vi "Measure Lowlevel.vi"(0 "VISA resource name":refnum<visa-resource-name>, 1 "Buffer Elements":string="READ", 5 "Timeout (10000 ms)":i32=10000 format="%#.6g", 7 "Buffer Name (defbuffer1)":string="defbuffer1", 9 "Function (0: Volts)":u16(ring) items=["Volts", "Current", "Digitize Voltage", "Digitize Current"], 11 "error in (no error)":errorcluster) -> (4 "VISA resource name out":refnum<visa-resource-name>, 6 "Data out":string, 15 "error out":errorcluster)   [LabVIEW 2022 SP3, in "Keithley 2450.lvlib"]
doc: "Measures data for voltage, current and resistance. \n\nBuffer Element can be a single parameter or multiple parameters.Parameters have to be separated by comma followed by space.(eg - READ, SEC, DATE)"
uses:
  Keithley 2450.lvlib
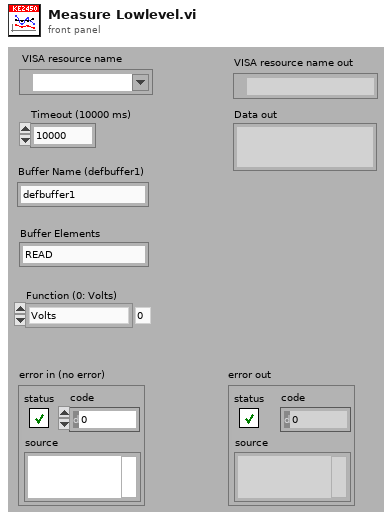
[diagram p1: front panel]
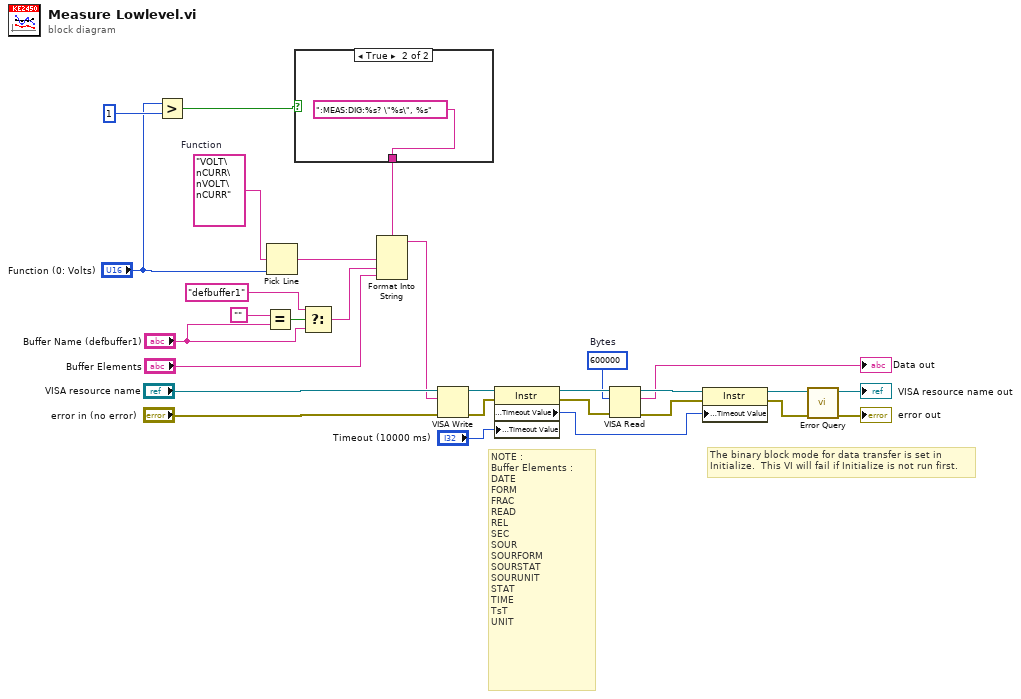
[diagram p0: block diagram]
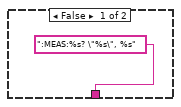
[diagram p2: hidden frame]
diagram:
  w9 = "VOLT\nCURR\nVOLT\nCURR"  # Function
  w20 = u32 600000  # Bytes
  # "NOTE :\nBuffer Elements :\nDATE\nFORM\nFRAC\nREAD\nREL\nSEC\nSOUR\nSOURFORM\nSOURSTAT\nSOURUNIT\nSTAT\nTIME\nTsT\nUNIT"
  # "The binary block mode for data transfer is set in Initialize.  This VI will fail if Initialize is not run first."
  n1 = Greater?(x="Function (0: Volts)", y=1) -> (0:w4:bool)
  n2 = Equal?(x="", y="Buffer Name (defbuffer1)") -> (x = y?=w16:bool)
  n3 = Pick Line(multi-line string=w9, line index="Function (0: Volts)") -> (output string=w8:string)  [unwired: 1 out]
  n4 = case shown="True" w4 {
    tunnel: [":MEAS:%s? \"%s\", %s" ("Fetch Measurement") ":MEAS:DIG:%s? \"%s\", %s" ("Fetch Measurement")] -> w3
    frame False {
    }
    frame True {
    }
  }
  n5 = Select(t="defbuffer1", s=w16, f="Buffer Name (defbuffer1)") -> (s? t:f=w7:string)
  n6 = Format Into String(format string=w3, w8, w7, "Buffer Elements") -> (resulting string=w6:string)  [unwired: 2 in, 1 out]
  n7 = VISA Write(VISA resource name="VISA resource name", write buffer=w6, error in (no error)="error in (no error)") -> (VISA resource name out=w18:refnum<visa-resource-name>, error out=w27:errorcluster)  [unwired: 1 out]
  n8 = property class="Instr"(reference=w18, error in=w27, "General Settings:Timeout Value"="Timeout (10000 ms)") -> (reference out=w26:refnum<visa-resource-name>, error out=w25:errorcluster, "General Settings:Timeout Value"=w21:u32)
  n9 = VISA Read(VISA resource name=w26, byte count=w20, error in (no error)=w25) -> (VISA resource name out=w23:refnum<visa-resource-name>, read buffer=→"Data out":string, error out=w22:errorcluster)  [unwired: 1 out]
  n10 = property class="Instr"(reference=w23, error in=w22, "General Settings:Timeout Value"=w21) -> (reference out=w13:refnum<visa-resource-name>, error out=w11:errorcluster)
  n11 = call "Error Query.vi"("error in (no error)"=w11, "VISA resource name"=w13) -> ("error out"=→"error out":errorcluster, "VISA resource name out"=→"VISA resource name out":refnum<visa-resource-name>)  [unwired: 8 out]
